vi "Get Paths and Names (SubVI).vi"(11 "Custom Device Folder":path) -> (0 "Custom Device Library":path, 1 "Custom Device Project":path, 2 "Custom Device Name":string, 3 "Custom Device Folder":path)   [LabVIEW 2010]
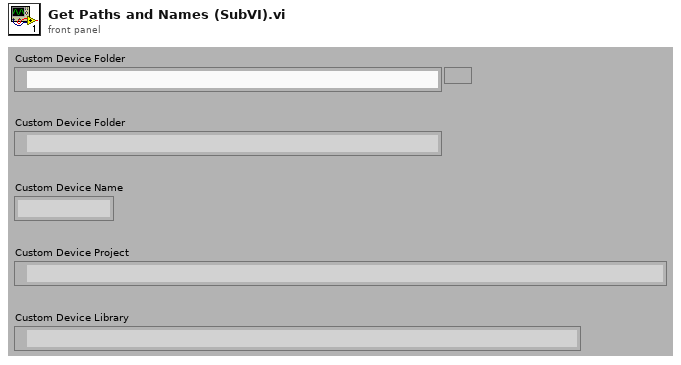
[diagram p1: front panel]
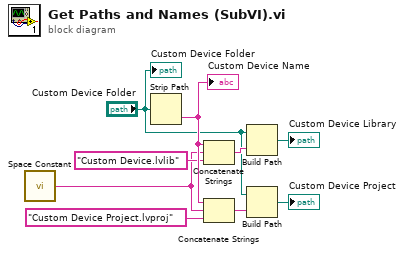
[diagram p0: block diagram]
diagram:
  n1 = call <vilib>:"Space Constant.vi"() -> ("String"=w1:string)
  n2 = Strip Path(path="Custom Device Folder") -> (name=w7:string)  [unwired: 1 out]
  "Custom Device Name" <- w7
  n3 = Concatenate Strings(w7, w1, "Custom Device.lvlib" ("string")) -> (w8:string)
  n4 = Concatenate Strings(w7, w1, "Custom Device Project.lvproj" ("string")) -> (w6:string)
  n5 = Build Path(base path="Custom Device Folder", name or relative path=w8) -> (appended path=→"Custom Device Library":path)
  n6 = Build Path(base path="Custom Device Folder", name or relative path=w6) -> (appended path=→"Custom Device Project":path)
  "Custom Device Folder" <- "Custom Device Folder"
